vi "UnitTest.vi"() -> ()   [LabVIEW 2019, in "DriveOld.lvlib" / "Drive.lvclass"]
uses:
  Drive.lvclass
panel:
  in  "WPI?":bool
  in  "stop":bool
  out "Right":dbl(slide) scale=-2.0..2.0
  out "Left":dbl(slide) scale=-2.0..2.0
  in  "Right":dbl(slide) min=-1.0 max=1.0 step=0.1 scale=-1.0..1.0
  in  "Forward":dbl(slide) min=-1.0 max=1.0 step=0.1 scale=-1.0..1.0
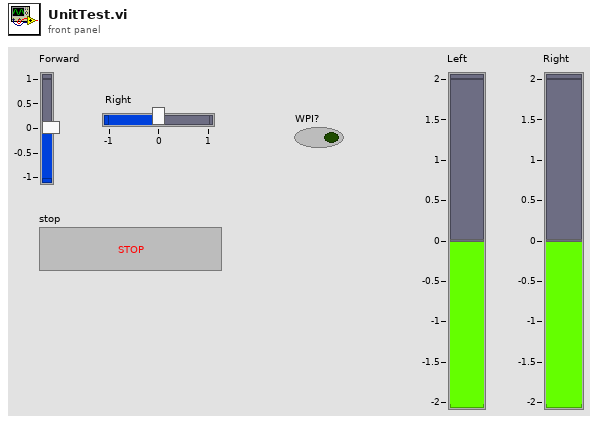
[diagram p1: front panel]
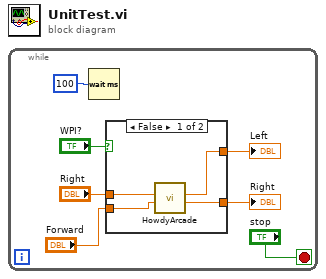
[diagram p0: block diagram]
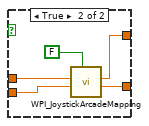
[diagram p2: hidden frame]
diagram:
  n1 = while {
    stop <- "stop" stop-if-true
    n2 = Wait (ms)(milliseconds to wait=u32 100) -> ()  [unwired: 1 out]
    n3 = case shown="False" "WPI?" {
      tunnel: "Right" -> [w11 w12]
      tunnel: "Forward" -> [w9 w16]
      tunnel: [w10 w15] -> w3
      tunnel: [w8 w14] -> w2
      frame False {
        n4 = call "HowdyArcade.vi"("forward"=w9, "right"=w11) -> ("right_wheel"=w8:dbl, "left_wheel"=w10:dbl)  [unwired: 8 in]
      }
      frame True {
        n5 = call <vilib>:"WPI_JoystickArcadeMapping.vi"("Square Inputs"=FALSE, "Y axis value"=w16, "X axis value"=w12) -> ("Right Motor Value"=w14:dbl, "Left Motor Value"=w15:dbl)  [unwired: 7 in]
      }
    }
    "Left" <- w3
    "Right" <- w2
  }
